vi "Start.vi"(8 "error in (no error)":errorcluster, 11 "CodeCoverage in":refnum<class "Code Coverage.lvclass">) -> (0 "error out":errorcluster, 3 "CodeCoverage out":refnum<class "Code Coverage.lvclass">)   [LabVIEW 2017, in "Code Coverage.lvclass"]
doc: "Start/Continue measuring code coverage."
uses:
  Code Coverage.lvclass
  Code Coverage.lvclass/Code Coverage.ctl
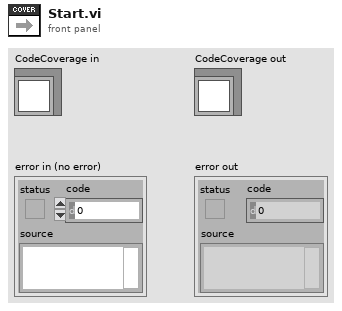
[diagram p1: front panel]
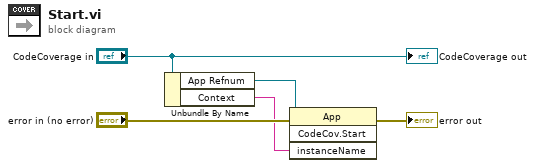
[diagram p0: block diagram]
diagram:
  n1 = Unbundle By Name("CodeCoverage in") -> ("App Refnum"=w3:refnum<vi>, "Context"=w1:string)
  n2 = invoke class="App" method="CodeCov.Start"(reference=w3, error in="error in (no error)", "instanceName"=w1) -> (error out=→"error out":errorcluster)  [unwired: 1 in, 3 out]
  "CodeCoverage out" <- "CodeCoverage in"
